vi "Value.vi"(8 "error in (no error)":errorcluster, 11 "Operator in":refnum<class "Operator.lvclass">) -> (0 "error out":errorcluster, 2 "Value":i64, 3 "Operator out":refnum<class "Operator.lvclass">)   [LabVIEW 2020, in "Operator.lvclass"]
uses:
  Operator.lvclass
  C:/dev/IlluminatedG/AdventOfCode/2021/source/Day 16/Part 1/Packet/Packet.lvclass
  Packet/Packet.lvclass
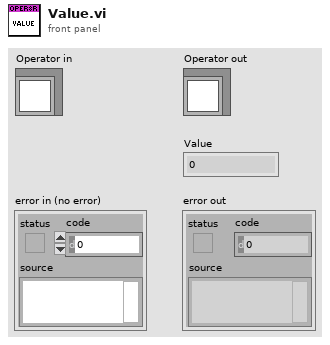
[diagram p1: front panel]
types:
  T1 = typedef "Type.ctl" = enum8{"Sum", "Product", "Minimum", "Maximum", "Literal", "Greater", "Less", "Equal"}
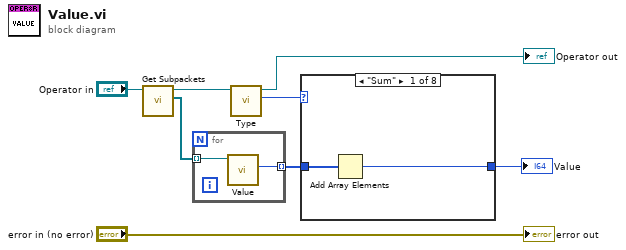
[diagram p0: block diagram]
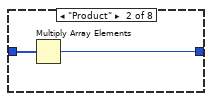
[diagram p2: hidden frame]
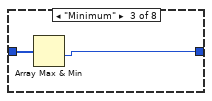
[diagram p3: hidden frame]
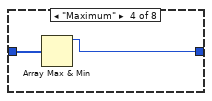
[diagram p4: hidden frame]
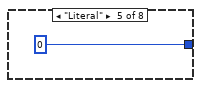
[diagram p5: hidden frame]
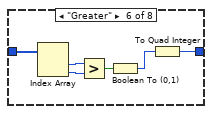
[diagram p6: hidden frame]
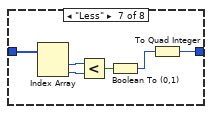
[diagram p7: hidden frame]
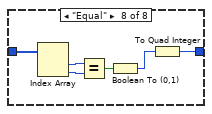
[diagram p8: hidden frame]
diagram:
  n1 = call-dynamic "Get Subpackets.vi"("Operator in"="Operator in") -> ("Subpackets"=w6:refnum<class "Packet.lvclass">[], "Operator out"=w5:refnum<class "Operator.lvclass">)  [unwired: 8 in, 1 out]
  n2 = for {
    tunnel: w6 -> [w10] mode=indexing
    tunnel: [w9] -> w3 mode=indexing
    n3 = call-dynamic "Value.vi"("Packet in"=w10) -> ("Value"=w9:i64)  [unwired: 8 in, 2 out]
  }
  n4 = call "Type.vi"("Packet in"=w5) -> ("Type"=w4:T1, "Packet out"=→"Operator out":refnum<class "Operator.lvclass">)  [unwired: 8 in, 1 out]
  n5 = case shown="\"Sum\"" w4 {
    tunnel: w3 -> [w12 w14 w16 w18 _ w25 w31 w37]
    tunnel: [w11 w13 w15 w17 i64 0 ("Value") w20 w26 w32] -> w2
    frame "Sum" {
      n6 = Add Array Elements(numeric array=w12) -> (sum=w11:i64)
    }
    frame "Product" {
      n7 = Multiply Array Elements(1:w14) -> (0:w13:i64)
    }
    frame "Minimum" {
      n8 = Array Max & Min(array=w16) -> (min value=w15:i64)  [unwired: 3 out]
    }
    frame "Maximum" {
      n9 = Array Max & Min(array=w18) -> (max value=w17:i64)  [unwired: 3 out]
    }
    frame "Literal" {
    }
    frame "Greater" {
      n10 = Index Array(array=w25) -> (element #1=w24:i64, element #2=w23:i64)  [unwired: 2 in]
      n11 = Greater?(x=w24, y=w23) -> (0:w22:bool)
      n12 = Boolean To (0,1)(Boolean=w22) -> (0, 1=w21:i16)
      n13 = To Quad Integer(1:w21) -> (0:w20:i64)
    }
    frame "Less" {
      n14 = Index Array(array=w31) -> (element #1=w30:i64, element #2=w29:i64)  [unwired: 2 in]
      n15 = Less?(x=w30, y=w29) -> (x < y?=w28:bool)
      n16 = Boolean To (0,1)(Boolean=w28) -> (0, 1=w27:i16)
      n17 = To Quad Integer(1:w27) -> (0:w26:i64)
    }
    frame "Equal" {
      n18 = Index Array(array=w37) -> (element #1=w36:i64, element #2=w35:i64)  [unwired: 2 in]
      n19 = Equal?(x=w36, y=w35) -> (x = y?=w34:bool)
      n20 = Boolean To (0,1)(Boolean=w34) -> (0, 1=w33:i16)
      n21 = To Quad Integer(1:w33) -> (0:w32:i64)
    }
  }
  "Value" <- w2
  "error out" <- "error in (no error)"
